vi "Demo_Guide.vi"(6 "Time In":i32, 8 "Temperature Sync":i32, 10 "Duration -1":i32, 11 "TempGuide":bool) -> (2 "Output array":dbl[](array[numeric]), 4 "Time out":i32)   [LabVIEW 2014]
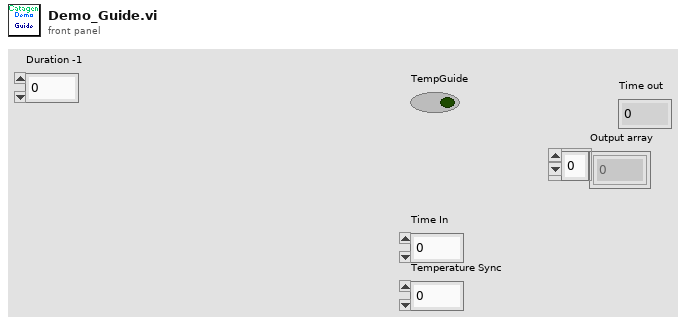
[diagram p1: front panel]
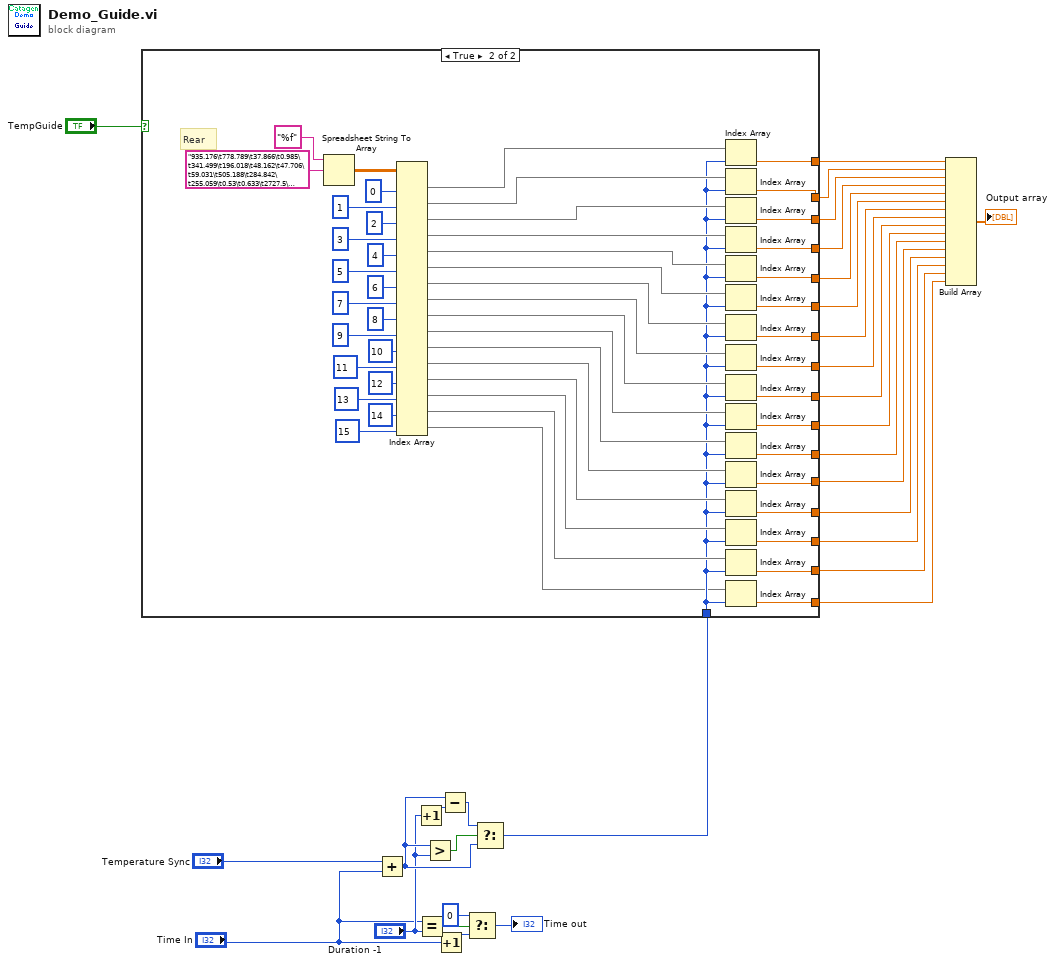
[diagram p0: block diagram]
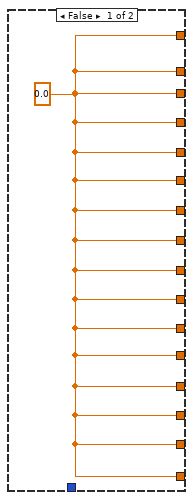
[diagram p2: hidden frame]
diagram:
  n1 = Add(x="Temperature Sync", y="Time In") -> (x+y=w23:i32)
  n2 = Increment(x="Duration -1") -> (x+1=w22:i32)
  n3 = Equal?(x="Time In", y="Duration -1") -> (x = y?=w28:bool)
  n4 = Greater?(x=w23, y="Duration -1") -> (0:w25:bool)
  n5 = Increment(x="Time In") -> (x+1=w26:i32)
  n6 = Subtract(x=w23, y=w22) -> (x-y=w24:i32)
  n7 = Select(t=0, s=w28, f=w26) -> (s? t:f=→"Time out":i32)
  n8 = Select(t=w24, s=w25, f=w23) -> (s? t:f=w20:i32)
  n9 = case shown="True" "TempGuide" {
    tunnel: w20 -> [_ w34]
    tunnel: [w31 w76] -> w17
    tunnel: [w31 w77] -> w16
    tunnel: [w31 w79] -> w15
    tunnel: [w31 w78] -> w14
    tunnel: [w31 w51] -> w13
    tunnel: [w31 w50] -> w12
    tunnel: [w31 w49] -> w11
    tunnel: [w31 w48] -> w10
    tunnel: [w31 w47] -> w9
    tunnel: [w31 w46] -> w8
    tunnel: [w31 w45] -> w7
    tunnel: [w31 w44] -> w6
    tunnel: [w31 w43] -> w5
    tunnel: [w31 w42] -> w4
    tunnel: [w31 w41] -> w3
    tunnel: [w31 w33] -> w1
    frame False {
      w31 = 0.0
    }
    frame True {
      # "Rear"
      n10 = Spreadsheet String To Array(format string="%f", spreadsheet string="935.176\t778.789\t37.866\t0.985\t341.499\t196.018\t48.162\t47.706\t59.031\t505.188\t284.842\t255.059\t0.53\t0.633\t2727.5\t2977.7\n935.434\t778.252\t38.467\t0.997\t340.846\t196.191\t48.175\t47.743\t59.015\t505.071\t284.806\t255.227\t0.532\t0.62\t2756.5\t2999.7\n935.176\t778.107\t38.566\t0.988\t341.235\t196.029\t48.184\t47.746\t58.786\t505.087\t284.824\t255.263\t0.53\t0.62\t2702.8\t2938.8\n935.434\t778.905\t38.245\t0.987\t341.412\t196.36\t48.191\t47.765\t58.934\t505.096\t284.8\t255.602\t0.526\t0.635\t2694.5\t2925.3\n935.176\t779.117\t38.779\t0.997\t341.284\t196.445\t48.218\t47.771\t59.115\t505.004\t284.775\t255.628\t0.526\t0.64\t2737.5\t2932.6\n935.434\t779.884\t37.804\t0.992\t341.638\t196.151\t48.197\t47.739\t58.988\t504.89\t284.78\t255.722\t0.524\t0.643\t2626.8\t3000.6\n935.176\t779.693\t37.802\t0.992\t341.083\t196.211\t48.212\t47.741\t58.928\t504.919\t284.767\t255.653\t0.521\t0.63\t2613.1\t2956.8\n935.434\t779.335\t37.403\t0.986\t341.606\t196.297\t48.178\t47.779\t59.016\t504.95\t284.74\t255.751\t0.517\t0.632\t2680.7\t2958.7\n935.64\t779.428\t37.495\t0.989\t341.597\t196.192\t48.19\t47.74\t58.892\t504.848\t284.733\t255.92\t0.515\t0.641\t2623\t3018.3\n935.712\t779.671\t37.594\t0.999\t341.111\t196.268\t48.207\t47.743\t58.728\t504.8\t284.745\t256.3\t0.513\t0.623\t2771.4\t2935.1\n935.858\t779.101\t37.109\t0.992\t341.339\t196.348\t48.172\t47.731\t58.819\t504.773\t284.695\t256.384\t0.512\t0.626\t2772\t2958.5\n935.743\t779.17\t37.125\t0.99\t341.362\t196.519\t48.195\t47.708\t58.782\t504.73\t284.708\t256.344\t0.513\t0.62\t2636.7\t3009.5\n935.765\t778.713\t38.036\t0.989\t341.21\t196.521\t48.207\t47.719\t58.66\t504.715\t284.725\t256.66\t0.513\t0.619\t2747.2\t3032\n935.972\t778.864\t38.515\t0.988\t340.951\t196.54\t48.169\t47.735\t58.542\t504.645\t284.706\t256.678\t0.512\t0.619\t2682.7\t3016.1\n935.874\t779.25\t37.723\t0.994\t341.447\t196.465\t48.17\t47.743\t58.76\t504.667\t284.695\t256.889\t0.512\t0.619\t2625.8\t2982.2\n936.057\t779.259\t37.612\t0.99\t341.131\t196.459\t48.171\t47.755\t58.81\t504.647\t284.673\t257.047\t0.51\t0.623\t2649.4\t2974.1\n936.243\t779.468\t38.081\t0.994\t341.192\t196.602\t48.203\t47.701\t58.791\t504.657\t284.648\t257.256\t0.509\t0.632\t2505.5\t3001.9\n936.411\t779.84\t37.666\t0.989\t340.827\t196.509\t48.19\t47.71\t58.85\t504.637\t284.652\t257.29\t0.512\t0.638\t2624.9\t2976.8\n936.475\t780.236\t38.135\t0.988\t340.804\t196.733\t48.209\t47.731\t58.893\t504.593\t284.644\t257.18\t0.51\t0.632\t2761.7\t2970.1\n936.697\t779.877\t37.978\t0.994\t340.784\t196.556\t48.191\t47.729\t58.931\t504.611\t284.654\t257.154\t0.512\t0.624\t2620.9\t2979.8\n936.757\t780.549\t38.359\t0.992\t341.119\t196.48\t48.201\t47.731\t59.047\t504.58\t284.66\t257.294\t0.517\t0.62\t2681.6\t2985.4\n936.612\t779.944\t39.107\t0.99\t341.468\t196.699\t48.2\t47.727\t58.927\t504.5\t284.635\t257.137\t0.514\t0.623\t2643.7\t2937.4\n936.708\t779.812\t38.107\t0.989\t341.014\t196.659\t48.214\t47.741\t59.091\t504.54\t284.632\t257.045\t0.513\t0.622\t2663\t2914.5\n936.651\t779.851\t38.921\t0.995\t341.35\t196.461\t48.218\t47.715\t59.127\t504.493\t284.629\t257.302\t0.513\t0.636\t2701.7\t2960\n936.764\t779.899\t38.331\t0.983\t341.498\t196.74\t48.197\t47.743\t59.208\t504.541\t284.65\t257.357\t0.517\t0.627\t2652.9\t2997\n936.692\t779.549\t39.035\t0.994\t341.688\t196.763\t48.196\t47.7\t58.976\t504.559\t284.641\t257.557\t0.513\t0.622\t2723.6\t2990.5\n936.614\t779.995\t38.25\t0.996\t341.694\t196.763\t48.222\t47.746\t59.211\t504.483\t284.641\t257.434\t0.514\t0.635\t2685.6\t2952.3\n936.672\t779.935\t37.552\t0.995\t341.024\t196.83\t48.195\t47.718\t59.122\t504.372\t284.633\t257.367\t0.513\t0.636\t2572.6\t2963.5\n936.619\t780.039\t37.651\t0.989\t341.505\t196.846\t48.206\t47.742\t59.303\t504.484\t284.641\t257.63\t0.515\t0.625\t2558.5\t2958.3\n936.748\t779.333\t37.213\t0.986\t341.04\t196.743\t48.177\t47.723\t59.399\t504.427\t284.621\t257.509\t0.514\t0.621\t2535.8\t2947.8\n936.69\t779.516\t36.632\t0.981\t340.992\t196.95\t48.198\t47.782\t59.218\t504.452\t284.632\t257.359\t0.515\t0.621\t2448.2\t2963.4\n936.626\t780.187\t37.573\t0.983\t341.155\t196.815\t48.18\t47.727\t59.339\t504.475\t284.63\t257.436\t0.513\t0.623\t2589.1\t2934.7\n936.726\t780.537\t37.902\t0.995\t341.73\t196.838\t48.171\t47.714\t59.205\t504.443\t284.622\t257.429\t0.51\t0.627\t2655.8\t2940.8\n936.752\t780.615\t37.787\t0.99\t341.327\t196.923\t48.202\t47.742\t59.187\t504.424\t284.614\t257.838\t0.511\t0.626\t2617.5\t2982.3\n936.772\t780.54\t38.356\t0.987\t341.334\t196.973\t48.212\t47.752\t59.213\t504.417\t284.613\t258.046\t0.513\t0.622\t2727.2\t2974\n937.007\t780.465\t37.779\t0.992\t341.31\t196.899\t48.186\t47.724\t59.257\t504.423\t284.62\t257.984\t0.511\t0.634\t2637.1\t2999.7\n937.055\t780.807\t37.614\t0.985\t341.385\t196.94\t48.178\t47.741\t59.384\t504.521\t284.597\t257.855\t0.514\t0.633\t2571.3\t3042.2\n937.02\t780.855\t37.301\t0.992\t341.298\t197.071\t48.198\t47.701\t59.341\t504.369\t284.596\t257.945\t0.512\t0.622\t2544.2\t2995.4\n937.094\t780.848\t37.911\t0.987\t341.46\t196.881\t48.188\t47.737\t59.313\t504.384\t284.615\t257.851\t0.512\t0.623\t2626\t2995.8\n937.026\t780.395\t38.179\t0.989\t341.623\t196.87\t48.196\t47.729\t59.422\t504.472\t284.584\t257.746\t0.51\t0.618\t2598.3\t2939.6\n937.101\t780.423\t38.211\t0.994\t341.558\t196.823\t48.184\t47.742\t59.347\t504.379\t284.627\t257.63\t0.513\t0.62\t2544.1\t2960.9\n937.03\t780.992\t38.9\t0.986\t341.345\t197.028\t48.196\t47.774\t59.412\t504.415\t284.614\t257.515\t0.513\t0.614\t2661.5\t2997.2\n937.159\t780.887\t38.517\t0.994\t341.798\t196.932\t48.175\t47.721\t59.507\t504.381\t284.599\t257.488\t0.511\t0.608\t2528.8\t2987.1\n937.12\t781.05\t38.663\t0.997\t341.212\t197.087\t48.186\t47.766\t59.535\t504.376\t284.594\t257.426\t0.512\t0.616\t2551.8\t2995.5\n937.269\t781.228\t38.419\t0.999\t341.648\t197.056\t48.174\t47.73\t59.653\t504.351\t284.567\t257.554\t0.513\t0.618\t2589.3\t2975.3\n937.303\t780.409\t38.086\t0.99\t341.211\t196.796\t48.192\t47.757\t59.674\t504.39\t284.551\t257.68\t0.509\t0.627\t2585.4\t2965.8\n937.36\t779.985\t38.442\t0.995\t341.226\t196.76\t48.182\t47.761\t59.766\t504.358\t284.543\t257.603\t0.51\t0.631\t2472.3\t2957.6\n937.573\t780.222\t38.161\t0.983\t341.711\t197.024\t48.174\t47.737\t59.655\t504.36\t284.567\t258.008\t0.512\t0.628\t2558.6\t2962.8\n937.704\t780.195\t37.94\t0.994\t341.047\t197.123\t48.177\t47.757\t59.577\t504.34\t284.563\t257.954\t0.512\t0.624\t2583.1\t2933.9\n937.696\t780.091\t37.606\t0.983\t341.461\t197.041\t48.193\t47.76\t59.664\t504.45\t284.587\t257.942\t0.51\t0.616\t2590.3\t2950.7\n937.721\t780.573\t38.193\t0.995\t341.005\t197.113\t48.198\t47.747\t59.624\t504.339\t284.572\t257.958\t0.512\t0.619\t2641.5\t2964.8\n937.842\t780.283\t38.252\t0.99\t341.225\t197.035\t48.174\t47.753\t59.695\t504.38\t284.579\t257.894\t0.51\t0.627\t2587.8\t3001.6\n937.816\t780.437\t37.667\t0.989\t341.281\t197.086\t48.172\t47.741\t59.555\t504.344\t284.583\t257.773\t0.512\t0.624\t2556\t3014.1\n937.681\t780.377\t37.312\t0.997\t341.249\t197.121\t48.176\t47.732\t59.857\t504.368\t284.568\t257.792\t0.511\t0.613\t2559.6\t3012.2\n937.737\t780.527\t36.967\t0.997\t341.689\t197.046\t48.171\t47.773\t59.683\t504.311\t284.6\t257.965\t0.509\t0.618\t2637.1\t2964.3\n937.752\t780.411\t36.684\t0.987\t341.455\t197.105\t48.191\t47.744\t59.672\t504.405\t284.581\t258.405\t0.508\t0.628\t2598.6\t2973.4\n937.769\t780.343\t37.145\t0.988\t340.929\t197.024\t48.193\t47.771\t59.632\t504.235\t284.599\t258.602\t0.511\t0.628\t2564.2\t2998.3\n937.76\t780.58\t37.677\t0.995\t341.253\t196.93\t48.188\t47.768\t59.545\t504.3\t284.568\t258.497\t0.511\t0.622\t2517\t2981.5\n937.772\t780.846\t37.534\t0.995\t341.337\t196.882\t48.186\t47.726\t59.507\t504.364\t284.584\t258.571\t0.512\t0.616\t2595.5\t2966.3\n937.811\t780.699\t37.866\t0.989\t341.393\t196.97\t48.216\t47.687\t59.666\t504.292\t284.61\t258.424\t0.512\t0.609\t2634.1\t2979\n937.908\t780.907\t38\t0.989\t341.631\t196.95\t48.204\t47.727\t59.541\t504.313\t284.597\t258.407\t0.512\t0.602\t2611.7\t2989.4\n937.941\t781.142\t37.483\t0.994\t341.408\t196.868\t48.192\t47.748\t59.496\t504.33\t284.585\t258.369\t0.513\t0.614\t2627.8\t3032.4\n937.845\t781.4\t37.634\t0.994\t341.591\t197.055\t48.201\t47.695\t59.522\t504.248\t284.579\t258.571\t0.513\t0.616\t2642\t3043.8\n937.8\t781.521\t38.641\t0.985\t341.344\t197.084\t48.179\t47.733\t59.509\t504.244\t284.59\t258.667\t0.514\t0.612\t2549.4\t3059.8\n937.656\t781.383\t38.541\t0.997\t341.695\t196.836\t48.195\t47.772\t59.598\t504.257\t284.584\t258.66\t0.51\t0.617\t2488.4\t2970.6\n937.636\t781.045\t38.066\t0.989\t341.264\t197.122\t48.214\t47.771\t59.561\t504.276\t284.605\t258.611\t0.509\t0.637\t2535.2\t2968.8\n937.446\t780.651\t36.915\t0.988\t341.341\t197.157\t48.194\t47.763\t59.49\t504.268\t284.573\t258.404\t0.514\t0.626\t2615.9\t2985.9\n937.469\t780.413\t37.637\t0.988\t341.069\t197.239\t48.199\t47.701\t59.574\t504.263\t284.578\t258.149\t0.513\t0.611\t2619.5\t2986.6\n937.399\t780.169\t38.34\t0.994\t341.482\t197.296\t48.199\t47.732\t59.391\t504.301\t284.572\t258.001\t0.512\t0.609\t2681.3\t2955.8\n937.309\t780.134\t38.079\t1\t341.149\t196.956\t48.224\t47.751\t59.287\t504.279\t284.594\t257.942\t0.512\t0.617\t2624.3\t2944.1\n937.333\t780.942\t38.277\t0.994\t341.111\t197.071\t48.211\t47.706\t59.357\t504.331\t284.56\t257.807\t0.511\t0.62\t2661.7\t2946.6\n937.357\t780.895\t38.73\t0.987\t341.739\t197.173\t48.201\t47.696\t59.307\t504.253\t284.562\t257.71\t0.511\t0.629\t2656.5\t2952.7\n937.445\t780.892\t37.894\t0.995\t340.896\t197.423\t48.199\t47.751\t59.344\t504.174\t284.555\t257.661\t0.514\t0.625\t2679.8\t2983.6\n937.543\t781.456\t37.122\t0.99\t341.519\t197.465\t48.201\t47.762\t59.419\t504.136\t284.555\t257.784\t0.512\t0.619\t2588.4\t2958.6\n937.48\t781.71\t37.166\t0.988\t341.265\t197.368\t48.214\t47.745\t59.169\t504.238\t284.55\t257.656\t0.513\t0.636\t2607.1\t3012\n937.655\t781.467\t37.912\t0.995\t340.931\t197.523\t48.196\t47.725\t59.188\t504.166\t284.561\t257.795\t0.513\t0.633\t2621.8\t2979.9\n937.619\t780.81\t37.891\t0.986\t341.023\t197.314\t48.191\t47.779\t59.242\t504.216\t284.55\t258.035\t0.513\t0.626\t2565.1\t2978.1\n937.606\t780.328\t37.164\t0.995\t340.932\t197.405\t48.233\t47.722\t59.271\t504.328\t284.563\t257.911\t0.515\t0.628\t2693.5\t2965.4\n937.658\t779.994\t37.707\t0.986\t341.384\t197.431\t48.193\t47.734\t59.349\t504.335\t284.579\t257.843\t0.511\t0.623\t2545.2\t2931.6\n937.534\t780.267\t37.464\t0.99\t341.454\t197.426\t48.222\t47.762\t59.215\t504.216\t284.581\t257.773\t0.514\t0.633\t2524.1\t2972.7\n937.567\t780.458\t37.531\t0.985\t341.44\t197.467\t48.223\t47.725\t59.207\t504.277\t284.574\t258.091\t0.513\t0.624\t2522.2\t2941.1\n937.646\t780.773\t37.219\t0.995\t341.442\t197.379\t48.237\t47.718\t59.139\t504.228\t284.607\t258.153\t0.511\t0.629\t2540.1\t2940.8\n937.651\t781.274\t36.752\t0.995\t341.26\t197.506\t48.225\t47.721\t59.186\t504.331\t284.587\t258.043\t0.512\t0.634\t2601.6\t2953.6\n937.699\t781.018\t38.18\t0.989\t341.377\t197.467\t48.191\t47.727\t59.024\t504.211\t284.594\t257.883\t0.51\t0.635\t2590.3\t2943.3\n937.701\t780.593\t38.142\t0.997\t341.244\t197.575\t48.217\t47.723\t59.185\t504.223\t284.581\t257.763\t0.511\t0.64\t2614.5\t2947.6\n937.719\t780.421\t38.259\t0.986\t341.031\t197.563\t48.213\t47.712\t59.108\t504.161\t284.618\t257.648\t0.512\t0.631\t2677.2\t2982.5\n937.596\t780.075\t36.986\t0.997\t340.923\t197.635\t48.204\t47.707\t59.192\t504.222\t284.619\t257.45\t0.513\t0.611\t2569.2\t2996.8\n937.554\t779.775\t37.442\t0.994\t341.06\t197.652\t48.207\t47.697\t59.094\t504.23\t284.604\t257.267\t0.515\t0.612\t2594.2\t3005.4\n937.509\t780.979\t37.896\t0.995\t341.338\t197.378\t48.201\t47.717\t59.085\t504.196\t284.597\t257.105\t0.514\t0.614\t2577.7\t2957.9\n937.532\t780.825\t38.135\t0.989\t340.98\t197.389\t48.203\t47.715\t59.208\t504.195\t284.595\t257.11\t0.513\t0.619\t2536.6\t2955.9\n937.615\t780.618\t37.439\t0.986\t340.835\t197.445\t48.202\t47.694\t59.039\t504.204\t284.606\t257.519\t0.514\t0.628\t2586.1\t2943\n937.677\t780.587\t38.426\t0.984\t341.449\t197.433\t48.222\t47.697\t59.25\t504.219\t284.587\t257.534\t0.511\t0.635\t2747.8\t2937.6\n937.782\t780.726\t37.747\t0.994\t340.919\t197.741\t48.195\t47.691\t58.995\t504.185\t284.598\t257.402\t0.512\t0.639\t2651.6\t2987.2\n937.791\t780.43\t38.054\t0.997\t341.401\t197.576\t48.209\t47.681\t59.065\t504.15\t284.605\t257.283\t0.515\t0.631\t2662.9\t3018.5\n937.796\t780.552\t38.671\t0.989\t341.401\t197.576\t48.209\t47.681\t59.065\t504.15\t284.605\t257.283\t0.515\t0.629\t2697.6\t3062.8\n937.691\t780.597\t38.063\t0.986\t341.126\t197.781\t48.182\t47.664\t58.905\t504.062\t284.577\t257.494\t0.516\t0.611\t2689.8\t2987.8\n937.785\t780.816\t38.613\t0.986\t341.11\t197.645\t48.206\t47.695\t59.026\t504.09\t284.619\t257.434\t0.515\t0.615\t2614\t2950.1\n937.159\t781.143\t37.946\t0.992\t341.526\t197.645\t48.203\t47.663\t59.012\t504.186\t284.613\t257.473\t0.514\t0.627\t2480.3\t2970.3\n937.12\t780.967\t38.207\t0.995\t341.335\t197.702\t48.168\t47.708\t59.179\t504.064\t284.61\t257.687\t0.515\t0.623\t2580.7\t2969.6\n937.269\t781.26\t38.17\t0.99\t341.325\t197.608\t48.182\t47.673\t59.091\t504.177\t284.619\t258.063\t0.513\t0.626\t2654.2\t2948.3\n937.303\t780.828\t37.483\t0.992\t341.228\t197.789\t48.2\t47.657\t59.084\t504.295\t284.612\t257.96\t0.514\t0.627\t2594.1\t3022.5\n937.36\t780.177\t36.062\t0.995\t341.349\t197.7\t48.171\t47.677\t59.014\t504.174\t284.627\t258.215\t0.516\t0.622\t2555.8\t3019.9\n937.573\t779.438\t21.721\t1.005\t340.91\t197.833\t48.159\t47.681\t59.08\t504.151\t284.581\t258.081\t0.514\t0.63\t2674.2\t2989.4\n937.704\t758.069\t3.721\t0.979\t339.657\t197.822\t48.189\t47.655\t58.911\t504.138\t284.575\t257.31\t0.513\t0.627\t2612.8\t2964.6\n937.696\t730.56\t5.4\t1.238\t337.665\t197.783\t48.179\t47.659\t58.843\t504.355\t284.551\t256.325\t0.515\t0.626\t2627.8\t2973.5\n937.159\t699.619\t2.079\t1.237\t335.324\t197.609\t48.192\t47.694\t59.087\t504.637\t284.584\t255.187\t0.515\t0.624\t2635.4\t2976.6\n937.12\t670.705\t0\t1.237\t333.7\t197.341\t48.173\t47.671\t59.079\t504.726\t284.568\t253.796\t0.516\t0.615\t9326.2\t2929.9\n937.269\t645.13\t6.364\t1.237\t331.426\t197.082\t48.19\t47.674\t59.24\t504.866\t284.573\t252.393\t0.512\t0.629\t32491\t2969.1\n937.303\t621.932\t16.517\t1.237\t329.251\t196.706\t48.191\t47.676\t59.331\t505.052\t284.594\t251.049\t0.503\t0.671\t7495.4\t6736.9\n937.36\t635.732\t34.728\t1.027\t326.995\t196.257\t48.185\t47.706\t59.256\t505.104\t284.545\t250.028\t0.446\t1.887\t2032.3\t11231\n937.573\t694.328\t36.83\t0.996\t330.997\t195.89\t48.197\t47.651\t59.162\t504.95\t284.536\t249.854\t0.34\t5.045\t1612.9\t3709.6\n937.704\t727.285\t37.695\t0.997\t333.623\t195.547\t48.18\t47.711\t59.251\t504.88\t284.479\t249.998\t0.196\t8.02\t1564.8\t994.92\n937.696\t746.738\t36.83\t0.994\t335.551\t195.715\t48.183\t47.712\t59.076\t504.798\t284.498\t250.297\t0.112\t11.173\t1873.5\t486.76\n937.721\t758.753\t37.825\t0.994\t336.89\t195.663\t48.188\t47.712\t59.078\t504.673\t284.453\t250.507\t0.077\t13.704\t3312.9\t338.29\n937.842\t765.909\t38.136\t0.983\t337.477\t195.365\t48.184\t47.691\t58.884\t504.637\t284.421\t250.662\t0.058\t15.819\t3307.2\t539.28\n937.816\t769.975\t38.145\t0.988\t338.673\t195.259\t48.194\t47.723\t59.095\t504.555\t284.41\t251.002\t0.299\t15.023\t3140.4\t3002.4\n937.681\t772.961\t39.008\t0.993\t339.377\t195.639\t48.198\t47.703\t59.034\t504.512\t284.405\t251.149\t0.489\t5.843\t3136.1\t3151.7\n937.737\t774.589\t38.263\t0.992\t339.843\t195.46\t48.201\t47.655\t58.815\t504.458\t284.379\t251.527\t0.505\t1.532\t2892.7\t3093\n937.752\t775.599\t37.943\t0.992\t339.491\t195.416\t48.211\t47.665\t59.002\t504.237\t284.363\t252.142\t0.51\t1\t2920.6\t3076.7\n937.769\t776.637\t38.718\t0.998\t340.503\t195.806\t48.193\t47.71\t58.822\t504.2\t284.35\t252.274\t0.511\t0.855\t2957.2\t3003.9\n932.76\t777.454\t38.453\t0.994\t340.638\t195.624\t48.214\t47.695\t58.795\t504.193\t284.32\t252.42\t0.512\t0.788\t2799.8\t3022.6\n924.772\t777.587\t38.777\t0.985\t340.421\t195.646\t48.243\t47.681\t58.786\t504.208\t284.307\t252.575\t0.514\t0.738\t2670.9\t3049.3\n913.239\t777.866\t37.715\t0.992\t340.827\t195.735\t48.23\t47.686\t58.726\t504.086\t284.264\t253.02\t0.511\t0.695\t2628.8\t3007.2\n913.561\t778.427\t37.63\t0.984\t340.962\t195.901\t48.202\t47.68\t58.775\t504.029\t284.226\t253.095\t0.51\t0.669\t2636.1\t2999.1\n923.956\t779.027\t37.663\t0.986\t340.513\t195.813\t48.191\t47.684\t58.728\t503.937\t284.217\t253.709\t0.512\t0.653\t2663.3\t3003.6\n929.211\t778.621\t37.241\t0.998\t340.409\t195.881\t48.188\t47.671\t58.708\t503.904\t284.209\t254.071\t0.515\t0.638\t2564.1\t2948.6\n931.58\t778.208\t36.738\t0.997\t341.12\t195.932\t48.181\t47.716\t58.647\t503.9\t284.183\t254.297\t0.514\t0.646\t2716.8\t2936.7\n934.667\t778.126\t37.166\t0.997\t340.632\t195.861\t48.178\t47.654\t58.844\t503.878\t284.144\t254.266\t0.515\t0.645\t2663.5\t2993.6\n934.958\t778.184\t38.338\t1\t340.861\t195.809\t48.191\t47.697\t58.886\t503.801\t284.145\t254.267\t0.517\t0.628\t2653\t2994.5\n935.111\t778.733\t37.691\t0.997\t341.022\t195.919\t48.206\t47.664\t58.85\t503.722\t284.094\t254.217\t0.513\t0.624\t2584.5\t2989.4\n935.317\t779.304\t37.812\t0.996\t340.99\t196.014\t48.217\t47.684\t59.026\t503.766\t284.074\t254.239\t0.508\t0.625\t2720.6\t2969.1\n935.383\t779.167\t37.862\t0.994\t341.204\t195.932\t48.203\t47.681\t58.986\t503.703\t284.094\t254.329\t0.506\t0.639\t2666.1\t3016\n935.617\t778.76\t37.56\t0.995\t341.122\t195.924\t48.193\t47.712\t58.935\t503.637\t284.077\t254.347\t0.502\t0.637\t2698.3\t2991.4\n935.722\t779.114\t37.737\t0.996\t340.826\t195.942\t48.207\t47.706\t59.157\t503.703\t284.032\t254.517\t0.499\t0.649\t2720.1\t2981.8\n935.787\t778.716\t38.24\t0.995\t340.65\t195.942\t48.183\t47.635\t58.839\t503.603\t284.014\t254.707\t0.499\t0.648\t2718.4\t2980.9\n935.757\t778.623\t39.103\t0.997\t340.773\t196.06\t48.211\t47.663\t59.005\t503.63\t284.039\t254.635\t0.495\t0.643\t2611.5\t2936.3\n935.841\t778.38\t38.494\t0.989\t340.509\t196.073\t48.191\t47.702\t59.122\t503.568\t284.006\t254.69\t0.495\t0.643\t2654\t2963.1\n935.752\t778.915\t38.873\t0.992\t341.434\t196.283\t48.208\t47.693\t59.146\t503.584\t283.987\t254.647\t0.493\t0.637\t2638\t2953.3\n935.901\t778.686\t38.59\t0.991\t341.501\t196.175\t48.218\t47.71\t59.113\t503.543\t284\t254.586\t0.494\t0.637\t2686.8\t2926.5\n935.82\t779.333\t37.791\t0.996\t341.179\t196.58\t48.215\t47.666\t59.103\t503.537\t283.988\t254.819\t0.494\t0.64\t2665.7\t2940.5\n936.09\t779.776\t38.353\t0.995\t341.24\t196.388\t48.193\t47.703\t59.2\t503.525\t284.003\t255.218\t0.494\t0.65\t2629.8\t2961.5\n936.09\t779.468\t38.902\t0.997\t340.766\t196.392\t48.227\t47.715\t59.028\t503.495\t283.978\t255.516\t0.497\t0.648\t2664\t3017.1\n936.147\t779.085\t38.311\t0.995\t340.701\t196.58\t48.222\t47.716\t59.244\t503.386\t283.99\t255.513\t0.498\t0.634\t2675\t2998\n936.269\t778.961\t37.503\t0.986\t340.846\t196.568\t48.221\t47.707\t59.168\t503.483\t283.981\t255.505\t0.498\t0.634\t2646.5\t2988.9\n936.398\t779.428\t37.444\t0.991\t340.917\t196.292\t48.218\t47.7\t59.163\t503.356\t283.975\t255.715\t0.5\t0.643\t2672.6\t2972.8\n936.529\t779.226\t36.984\t0.994\t340.754\t196.3\t48.208\t47.737\t59.183\t503.495\t283.975\t255.967\t0.5\t0.634\t2615.1\t2987\n936.617\t778.995\t37.412\t0.995\t340.46\t196.486\t48.219\t47.678\t58.877\t503.486\t283.958\t255.837\t0.502\t0.63\t2634.9\t2973\n936.828\t779.321\t37.44\t0.987\t340.888\t196.508\t48.193\t47.738\t59.122\t503.441\t283.962\t255.957\t0.5\t0.63\t2703.4\t2958\n936.857\t779.719\t37.631\t0.998\t340.739\t196.457\t48.232\t47.725\t59.23\t503.446\t283.973\t256.298\t0.5\t0.632\t2695.8\t2972.8\n937.088\t779.724\t37.873\t0.989\t340.655\t196.426\t48.203\t47.708\t59.218\t503.479\t283.967\t256.283\t0.499\t0.632\t2730.9\t3004.2\n937.123\t780.264\t37.992\t0.994\t341.067\t196.539\t48.211\t47.717\t59.109\t503.425\t283.945\t256.532\t0.502\t0.628\t2670.5\t3016.3\n937.266\t780.302\t37.184\t0.998\t340.333\t196.497\t48.213\t47.712\t59.103\t503.338\t283.95\t256.641\t0.5\t0.632\t2577.4\t2982.7\n937.299\t780.011\t38.06\t0.997\t340.88\t196.561\t48.222\t47.717\t59.077\t503.397\t283.943\t256.554\t0.498\t0.643\t2783\t2983.8\n937.179\t780.1\t37.554\t0.984\t341.015\t196.489\t48.208\t47.669\t59.137\t503.374\t283.934\t256.725\t0.499\t0.645\t2690.2\t3021.2\n937.152\t780.222\t37.333\t0.997\t340.658\t196.493\t48.196\t47.685\t59.037\t503.387\t283.937\t256.716\t0.5\t0.624\t2746.2\t3019.7\n937.147\t779.592\t38.041\t0.989\t340.819\t196.483\t48.19\t47.676\t59.006\t503.433\t283.944\t256.785\t0.501\t0.617\t2666.1\t3053.9\n937.005\t779.641\t38.457\t0.999\t340.829\t196.68\t48.222\t47.72\t59.139\t503.436\t283.949\t257.097\t0.5\t0.612\t2717.7\t3009.4\n937.109\t779.22\t38.404\t0.997\t340.37\t196.631\t48.214\t47.695\t59.159\t503.363\t283.916\t257.014\t0.5\t0.62\t2700.7\t3001.6\n937.182\t779.367\t38.74\t0.991\t340.579\t196.583\t48.192\t47.72\t59.112\t503.385\t283.905\t257.023\t0.497\t0.626\t2604.3\t2931.7\n937.25\t780.055\t38.704\t0.986\t340.878\t196.734\t48.202\t47.726\t58.989\t503.417\t283.937\t257.464\t0.496\t0.643\t2657.9\t2977.5\n937.281\t780.444\t37.893\t0.986\t340.86\t196.849\t48.197\t47.722\t58.993\t503.411\t283.952\t257.361\t0.497\t0.64\t2597.5\t2970.8\n937.35\t780.499\t37.676\t0.985\t341.133\t196.559\t48.176\t47.722\t59.143\t503.442\t283.911\t257.29\t0.496\t0.631\t2555.2\t3014.5\n937.4\t780.551\t38.07\t0.996\t340.945\t196.545\t48.19\t47.728\t59.144\t503.416\t283.948\t257.452\t0.498\t0.625\t2646.5\t2997.3\n937.33\t780.035\t37.945\t0.992\t341.103\t196.538\t48.217\t47.68\t59.22\t503.41\t283.95\t257.573\t0.497\t0.627\t2768.9\t2982.7\n937.288\t780.109\t37.372\t0.988\t340.973\t196.539\t48.217\t47.698\t59.096\t503.433\t283.941\t257.583\t0.5\t0.621\t2677.5\t3017.4\n937.4\t779.676\t38.066\t0.998\t340.457\t196.762\t48.189\t47.695\t59.047\t503.408\t283.95\t257.615\t0.499\t0.622\t2594.2\t2988.6\n937.36\t780.035\t38.284\t1.004\t340.808\t196.642\t48.202\t47.695\t58.958\t503.472\t283.953\t257.49\t0.5\t0.625\t2613.1\t2987\n937.324\t780.101\t38.162\t0.989\t340.988\t196.829\t48.185\t47.722\t58.929\t503.425\t283.953\t257.484\t0.496\t0.618\t2650.8\t3012\n937.278\t780.194\t37.634\t0.99\t340.816\t196.906\t48.192\t47.679\t58.918\t503.398\t283.95\t257.883\t0.498\t0.622\t2645.3\t3002.2\n937.361\t780.669\t38.339\t0.997\t341.191\t196.793\t48.197\t47.715\t58.847\t503.47\t283.946\t258.173\t0.496\t0.625\t2627\t2951.3\n937.42\t780.516\t37.909\t1\t340.827\t196.854\t48.19\t47.713\t58.756\t503.372\t283.959\t258.165\t0.497\t0.641\t2560.5\t2971.8\n937.315\t780.583\t37.49\t0.992\t340.712\t197.006\t48.209\t47.669\t58.717\t503.385\t283.944\t258.187\t0.496\t0.647\t2532.7\t2990.7\n937.328\t780.528\t37.459\t0.995\t341.023\t196.881\t48.224\t47.735\t58.743\t503.407\t283.97\t258.052\t0.495\t0.639\t2789.6\t2990.7\n937.272\t780.276\t37.951\t0.998\t340.909\t196.958\t48.219\t47.665\t58.763\t503.388\t283.966\t258.094\t0.497\t0.63\t2728.7\t3013.6\n937.28\t779.637\t37.33\t0.998\t340.785\t196.903\t48.204\t47.694\t58.734\t503.305\t283.969\t258.284\t0.5\t0.62\t2610\t3023.6\n937.453\t780.073\t37.125\t0.99\t340.711\t196.881\t48.183\t47.723\t58.753\t503.362\t283.982\t258.13\t0.501\t0.62\t2751.2\t3014.8\n937.477\t780.286\t38.156\t0.998\t341.004\t196.821\t48.189\t47.734\t58.802\t503.404\t283.997\t257.975\t0.499\t0.618\t2676.8\t3046.5\n937.54\t780.564\t38.19\t0.997\t341.007\t196.874\t48.196\t47.705\t58.661\t503.47\t283.994\t258.024\t0.499\t0.615\t2689.2\t3027.4\n937.646\t780.604\t38.262\t0.994\t340.935\t196.802\t48.203\t47.702\t58.687\t503.384\t283.954\t258.05\t0.498\t0.629\t2678.8\t3024.3\n937.68\t780.601\t37.543\t0.992\t341.235\t196.788\t48.195\t47.692\t58.598\t503.374\t283.934\t258.008\t0.497\t0.63\t2707\t3047.7\n937.66\t780.536\t37.701\t0.997\t341.143\t196.949\t48.194\t47.714\t58.487\t503.352\t283.939\t257.902\t0.497\t0.626\t2632.8\t3035.3\n937.685\t780.73\t37.755\t0.997\t340.615\t197.062\t48.207\t47.72\t58.603\t503.378\t283.96\t257.89\t0.497\t0.628\t2581.5\t3021.9\n937.59\t780.439\t37.666\t0.992\t340.606\t197.027\t48.199\t47.704\t58.768\t503.349\t283.957\t257.878\t0.497\t0.637\t2542\t2972.6\n937.554\t780.055\t37.4\t0.997\t340.521\t197.126\t48.226\t47.695\t58.793\t503.418\t283.962\t257.88\t0.496\t0.649\t2627.7\t2997.6\n937.421\t779.622\t37.644\t0.992\t340.694\t196.903\t48.197\t47.708\t58.669\t503.301\t283.942\t258.137\t0.497\t0.638\t2651.9\t2980.7\n937.472\t779.212\t37.919\t0.999\t341.018\t197.108\t48.18\t47.719\t58.871\t503.397\t283.951\t258.114\t0.496\t0.62\t2641.7\t2981.6\n937.522\t779.257\t38.477\t0.995\t340.542\t197.066\t48.201\t47.73\t58.843\t503.382\t283.96\t257.937\t0.498\t0.627\t2680.2\t2979.4\n937.431\t779.93\t38.552\t0.984\t340.768\t197.072\t48.207\t47.727\t58.634\t503.345\t283.944\t257.834\t0.496\t0.634\t2609.1\t2963.6\n937.544\t780.57\t38.749\t0.989\t340.776\t197.116\t48.208\t47.731\t58.638\t503.351\t283.935\t258.05\t0.497\t0.642\t2553.8\t3017.4\n937.866\t780.205\t38.061\t0.993\t340.964\t197.132\t48.184\t47.685\t58.565\t503.263\t283.941\t257.945\t0.498\t0.633\t2532.6\t3045.4\n937.965\t780.324\t38.387\t0.995\t340.465\t197.059\t48.195\t47.668\t58.719\t503.333\t283.922\t258.052\t0.496\t0.623\t2615.4\t2986.2\n938.058\t780.139\t38.573\t0.997\t340.75\t197.24\t48.216\t47.645\t58.733\t503.408\t283.938\t258.305\t0.496\t0.635\t2630.6\t2973.8\n938.124\t780.104\t38.148\t0.994\t340.471\t197.237\t48.198\t47.713\t58.942\t503.335\t283.946\t258.463\t0.496\t0.637\t2658.5\t2955.3\n938.171\t780.104\t37.981\t0.995\t340.587\t197.203\t48.18\t47.683\t58.936\t503.221\t283.943\t258.744\t0.495\t0.637\t2652.6\t2922.5\n938.154\t780.128\t38.293\t1.001\t340.68\t197.171\t48.179\t47.701\t58.894\t503.318\t283.938\t258.736\t0.498\t0.64\t2629\t2916.6\n938.111\t779.891\t38.467\t0.998\t341.062\t197.046\t48.171\t47.719\t58.962\t503.216\t283.968\t258.479\t0.496\t0.641\t2638\t2939.8\n937.97\t779.689\t37.643\t0.993\t340.511\t197.024\t48.188\t47.684\t59.033\t503.336\t283.963\t258.285\t0.497\t0.641\t2642.6\t2962.3\n937.986\t780.02\t37.609\t0.994\t340.743\t197.021\t48.192\t47.671\t59.057\t503.34\t283.959\t258.322\t0.497\t0.64\t2613.9\t3040.1\n937.982\t779.773\t37.12\t0.989\t340.56\t197.026\t48.196\t47.724\t59.157\t503.352\t283.977\t258.187\t0.499\t0.627\t2623.8\t3035.9\n937.472\t780.132\t36.88\t0.989\t340.981\t196.954\t48.208\t47.683\t59.136\t503.322\t283.959\t257.91\t0.497\t0.626\t2607.9\t3005.8\n937.522\t780.278\t37.636\t0.993\t340.699\t196.972\t48.194\t47.7\t59.02\t503.329\t283.951\t257.862\t0.497\t0.636\t2637\t3004.2\n937.431\t780.266\t37.411\t0.989\t340.726\t197.044\t48.192\t47.711\t58.934\t503.331\t283.938\t258.148\t0.497\t0.643\t2558.2\t2977.2\n937.544\t780.266\t37.411\t0.989\t340.726\t197.044\t48.192\t47.711\t58.934\t503.331\t283.938\t258.148\t0.498\t0.644\t2641.1\t2996\n937.866\t779.733\t37.61\t0.989\t340.165\t196.91\t48.21\t47.728\t58.865\t503.281\t283.985\t258.342\t0.498\t0.627\t2737.2\t2984.1\n937.965\t779.887\t38.813\t0.994\t340.896\t197.017\t48.209\t47.703\t58.983\t503.332\t283.971\t258.582\t0.497\t0.618\t2651.5\t2980.3\n938.058\t780.007\t38.533\t0.991\t340.78\t196.909\t48.201\t47.723\t58.762\t503.307\t284.002\t258.719\t0.499\t0.627\t2580.1\t3030.3\n938.124\t780.272\t38.414\t0.986\t340.702\t197.068\t48.209\t47.681\t58.727\t503.309\t283.995\t258.807\t0.498\t0.627\t2641\t2986.7\n938.171\t780.238\t37.811\t1\t340.817\t197.048\t48.247\t47.691\t58.917\t503.299\t283.982\t258.913\t0.496\t0.636\t2619.5\t2986.8\n938.154\t779.884\t38.119\t0.994\t341.149\t196.857\t48.226\t47.689\t58.944\t503.304\t284\t259.12\t0.497\t0.637\t2593.3\t3019.6\n938.111\t780.103\t37.94\t0.987\t341.017\t196.94\t48.228\t47.699\t58.886\t503.272\t284.012\t259.15\t0.497\t0.629\t2622.3\t2983\n937.97\t780.473\t37.69\t0.997\t340.696\t196.955\t48.22\t47.703\t58.705\t503.331\t284.015\t259.093\t0.495\t0.635\t2637.3\t2944.5\n937.986\t780.7\t38.047\t0.996\t340.704\t197.075\t48.228\t47.714\t58.687\t503.313\t284.016\t259.004\t0.496\t0.639\t2651.8\t2934.5\n937.982\t780.57\t38.2\t0.988\t340.745\t197.274\t48.221\t47.685\t58.642\t503.276\t284.008\t258.888\t0.496\t0.638\t2662.9\t2929.9\n937.679\t780.668\t38.432\t0.987\t340.699\t197.026\t48.205\t47.686\t58.733\t503.3\t284.003\t258.652\t0.497\t0.629\t2641.2\t2953.5\n937.574\t780.81\t38.341\t0.997\t340.49\t197.027\t48.219\t47.709\t58.987\t503.261\t284.01\t258.677\t0.498\t0.636\t2687\t2949.7\n937.415\t780.686\t38.078\t0.987\t340.677\t197.001\t48.229\t47.684\t58.812\t503.23\t284.035\t258.623\t0.498\t0.642\t2706.4\t3026.7\n937.329\t780.278\t38.048\t0.995\t341.053\t197.31\t48.216\t47.691\t58.771\t503.313\t284.019\t258.422\t0.498\t0.626\t2808.9\t3063.7\n937.281\t779.859\t37.703\t0.996\t341.062\t197.245\t48.221\t47.679\t58.726\t503.282\t284.019\t258.649\t0.499\t0.628\t2690.9\t3024.9\n937.288\t780.523\t37.852\t0.989\t340.658\t196.943\t48.194\t47.712\t58.796\t503.303\t284\t258.572\t0.498\t0.639\t2705.1\t3007.3\n937.28\t780.835\t37.063\t0.995\t341.001\t197.106\t48.207\t47.67\t58.817\t503.32\t283.995\t258.539\t0.499\t0.642\t2584.4\t3061\n937.378\t780.687\t37.377\t0.995\t340.47\t196.919\t48.218\t47.67\t58.716\t503.251\t284.019\t258.472\t0.5\t0.625\t2528.5\t3032.1\n937.472\t780.963\t38.027\t0.994\t340.741\t196.966\t48.209\t47.652\t58.634\t503.297\t284.03\t258.54\t0.499\t0.621\t2618.2\t2988.4\n937.522\t780.819\t37.698\t0.995\t340.745\t197.038\t48.213\t47.648\t58.614\t503.366\t284.024\t258.535\t0.496\t0.622\t2680.5\t2938.2\n937.431\t780.902\t36.938\t0.989\t340.929\t196.954\t48.203\t47.69\t58.634\t503.392\t283.991\t258.492\t0.497\t0.632\t2676.2\t2926.7\n937.544\t781.04\t37.86\t0.994\t340.551\t196.998\t48.169\t47.68\t58.617\t503.305\t284.007\t258.639\t0.497\t0.637\t2688\t2989.5\n937.866\t780.863\t37.523\t0.998\t340.815\t197.018\t48.185\t47.694\t58.67\t503.246\t283.997\t258.51\t0.498\t0.631\t2689.3\t2992.9\n937.965\t780.606\t36.454\t0.997\t340.953\t197.104\t48.19\t47.707\t58.663\t503.259\t283.962\t258.331\t0.5\t0.625\t2566.6\t2995.7\n938.058\t779.715\t20.985\t1\t340.299\t197.202\t48.2\t47.7\t58.869\t503.301\t283.957\t258.262\t0.5\t0.625\t2621.6\t3032.3\n937.472\t757.72\t2.076\t0.978\t339.536\t197.02\t48.197\t47.693\t59.05\t503.359\t283.928\t257.468\t0.5\t0.622\t2706\t3070.6\n937.522\t729.923\t3.986\t1.238\t337.139\t196.876\t48.18\t47.647\t58.875\t503.51\t283.922\t256.471\t0.499\t0.621\t2528.8\t3021.8\n937.431\t698.461\t5.167\t1.237\t335.379\t196.718\t48.196\t47.68\t58.959\t503.685\t283.943\t255.345\t0.5\t0.629\t2525.5\t2990.2\n937.544\t669.672\t4.918\t1.237\t332.927\t196.751\t48.18\t47.697\t59.085\t503.848\t283.918\t254.011\t0.5\t0.628\t9480.3\t2945.3\n937.866\t643.975\t5.823\t1.236\t331.152\t196.485\t48.178\t47.672\t59.002\t503.995\t283.877\t252.747\t0.498\t0.634\t33177\t3016.2\n937.965\t620.889\t15.85\t1.235\t328.813\t196.065\t48.197\t47.694\t59.014\t504.083\t283.882\t251.446\t0.489\t0.663\t7645.4\t6720.2\n938.058\t633.622\t35.441\t1.02\t327.046\t195.468\t48.162\t47.66\t58.981\t504.176\t283.83\t250.288\t0.432\t1.878\t2077.5\t11293\n938.124\t692.704\t37.669\t1\t330.539\t194.921\t48.184\t47.644\t59.14\t504.141\t283.824\t250.068\t0.321\t5.116\t1631.8\t3747.3\n938.171\t726.459\t36.898\t0.997\t333.054\t194.571\t48.16\t47.645\t58.9\t503.975\t283.779\t250.118\t0.193\t8.196\t1569.9\t1068.2\n938.154\t746.551\t38.37\t0.997\t335.074\t194.479\t48.19\t47.676\t58.983\t503.989\t283.754\t250.227\t0.117\t11.136\t1878.2\t503.48\n938.111\t758.071\t38.542\t0.988\t336.375\t194.356\t48.18\t47.678\t59.067\t503.88\t283.753\t250.429\t0.075\t13.534\t3301.4\t336.55\n937.97\t765.35\t38.268\t0.993\t336.914\t194.489\t48.172\t47.661\t58.888\t503.789\t283.68\t250.636\t0.058\t15.686\t3260.8\t532.65\n937.986\t770.2\t38.24\t0.994\t338.245\t194.629\t48.163\t47.658\t58.97\t503.633\t283.676\t250.768\t0.304\t14.89\t3110.3\t2990.6\n937.982\t772.699\t38.378\t0.994\t338.388\t194.541\t48.163\t47.698\t59.061\t503.706\t283.665\t250.929\t0.469\t5.749\t3137.6\t3091.6\n937.769\t774.724\t38.531\t0.989\t338.846\t194.731\t48.172\t47.699\t58.853\t503.61\t283.629\t251.062\t0.484\t1.579\t3033.7\t3066\n932.76\t775.825\t38.971\t0.989\t339.704\t194.658\t48.193\t47.694\t58.952\t503.514\t283.628\t251.331\t0.491\t1.026\t2949.9\t3064.3\n924.772\t776.957\t39.041\t0.992\t339.623\t194.896\t48.16\t47.694\t58.916\t503.431\t283.571\t251.49\t0.494\t0.869\t2741.6\t3094.7\n913.239\t777.116\t38.531\t0.985\t340.214\t194.969\t48.135\t47.7\t59.019\t503.46\t283.546\t251.654\t0.498\t0.787\t2739.4\t3097.1\n913.561\t777.414\t38.256\t1\t339.978\t195.087\t48.159\t47.643\t58.899\t503.378\t283.527\t251.884\t0.495\t0.721\t2669.7\t3056.6\n923.956\t777.432\t37.841\t0.997\t340.017\t195.114\t48.159\t47.68\t58.925\t503.281\t283.505\t252.088\t0.494\t0.694\t2686.6\t2998.6\n929.211\t777.877\t37.393\t0.998\t340.097\t195.203\t48.195\t47.685\t58.915\t503.24\t283.489\t252.367\t0.494\t0.678\t2689.6\t3014.3\n931.58\t777.597\t37.61\t0.987\t340.136\t195.136\t48.162\t47.667\t58.868\t503.19\t283.481\t252.922\t0.495\t0.661\t2636.1\t2994.1\n934.667\t777.666\t37.938\t0.998\t340.299\t195.262\t48.172\t47.653\t58.686\t503.145\t283.46\t253.022\t0.496\t0.653\t2638.2\t2946.3\n934.958\t777.849\t37.39\t0.995\t340.087\t195.229\t48.165\t47.65\t58.663\t503.045\t283.456\t253.32\t0.499\t0.653\t2662.1\t2973.1\n934.274\t778.329\t37.766\t0.993\t339.98\t195.138\t48.155\t47.663\t58.693\t503.035\t283.429\t253.617\t0.498\t0.644\t2635.5\t2958.5\n934.593\t778.263\t37.755\t1\t340.165\t195.109\t48.167\t47.629\t58.608\t502.979\t283.404\t253.91\t0.497\t0.639\t2642.6\t2946.5\n934.69\t778.49\t39.043\t0.99\t340.572\t195.229\t48.187\t47.669\t58.758\t502.981\t283.433\t253.984\t0.493\t0.642\t2656\t2963.2\n935.022\t778.284\t38.297\t1\t340.334\t195.405\t48.16\t47.652\t58.77\t502.972\t283.383\t254.288\t0.49\t0.646\t2757.4\t2975.6\n935.07\t778.707\t37.924\t0.983\t340.496\t195.491\t48.156\t47.6\t58.658\t502.96\t283.394\t254.419\t0.487\t0.644\t2832.3\t3000.5\n935.224\t778.699\t37.687\t0.995\t340.439\t195.3\t48.169\t47.658\t58.754\t502.852\t283.377\t254.9\t0.486\t0.649\t2853.6\t2996.7\n935.524\t778.985\t38.446\t0.989\t340.32\t195.293\t48.159\t47.643\t58.541\t502.9\t283.379\t255.06\t0.483\t0.648\t2647.2\t2992.1\n935.611\t778.296\t38.62\t0.994\t340.443\t195.297\t48.152\t47.673\t58.59\t502.807\t283.367\t255.138\t0.484\t0.653\t2593.9\t3010.4\n935.855\t778.336\t38.702\t0.988\t340.128\t195.312\t48.151\t47.681\t58.553\t502.79\t283.356\t255.263\t0.48\t0.638\t2671.3\t2947.2\n935.932\t778.323\t38.287\t0.997\t340.169\t195.392\t48.142\t47.649\t58.599\t502.74\t283.347\t255.319\t0.477\t0.638\t2681.4\t2943.3\n936.126\t778.089\t38.26\t1.005\t340.634\t195.138\t48.142\t47.669\t58.556\t502.716\t283.343\t255.545\t0.476\t0.642\t2626.2\t2980.3\n") -> (array=w82:dbl[][])  [unwired: 2 in]
      n11 = Index Array(array=w82, index (col) #1=0 ("disabled index (col)"), index (col) #2=1 ("disabled index (col)"), index (col) #3=2 ("index (col)"), index (col) #4=3 ("index (col)"), index (col) #5=4 ("index (col)"), index (col) #6=5 ("index (col)"), index (col) #7=6 ("index (col)"), index (col) #8=7 ("index (col)"), index (col) #9=8 ("index (col)"), index (col) #10=9 ("index (col)"), index (col) #11=10 ("index (col)"), index (col) #12=11 ("index (col)"), index (col) #13=12 ("index (col)"), index (col) #14=13 ("index (col)"), index (col) #15=14 ("index (col)"), index (col) #16=15 ("index (col)")) -> (element #1=w74:dbl[], element #2=w73:dbl[], element #3=w64:dbl[], element #4=w63:dbl[], element #5=w62:dbl[], element #6=w61:dbl[], element #7=w60:dbl[], element #8=w59:dbl[], element #9=w58:dbl[], element #10=w57:dbl[], element #11=w56:dbl[], element #12=w55:dbl[], element #13=w54:dbl[], element #14=w53:dbl[], element #15=w52:dbl[], element #16=w32:dbl[])  [unwired: 16 in]
      n12 = Index Array(array=w74, index=w34) -> (element=w76:dbl)
      n13 = Index Array(array=w73, index=w34) -> (element=w77:dbl)
      n14 = Index Array(array=w64, index=w34) -> (element=w79:dbl)
      n15 = Index Array(array=w63, index=w34) -> (element=w78:dbl)
      n16 = Index Array(array=w62, index=w34) -> (element=w51:dbl)
      n17 = Index Array(array=w61, index=w34) -> (element=w50:dbl)
      n18 = Index Array(array=w60, index=w34) -> (element=w49:dbl)
      n19 = Index Array(array=w59, index=w34) -> (element=w48:dbl)
      n20 = Index Array(array=w58, index=w34) -> (element=w47:dbl)
      n21 = Index Array(array=w57, index=w34) -> (element=w46:dbl)
      n22 = Index Array(array=w56, index=w34) -> (element=w45:dbl)
      n23 = Index Array(array=w55, index=w34) -> (element=w44:dbl)
      n24 = Index Array(array=w54, index=w34) -> (element=w43:dbl)
      n25 = Index Array(array=w53, index=w34) -> (element=w42:dbl)
      n26 = Index Array(array=w52, index=w34) -> (element=w41:dbl)
      n27 = Index Array(array=w32, index=w34) -> (element=w33:dbl)
    }
  }
  n28 = Build Array(w17, w16, w15, w14, w13, w12, w11, w10, w9, w8, w7, w6, w5, w4, w3, w1) -> (→"Output array":dbl[])
